vi "系统设置.vi"() -> ()   [LabVIEW 2016]
uses:
  <vilib>/Utility/miscctls.llb/LVPointTypeDef.ctl
  <userlib>/_SmartBalloon/Balloon Generic/Aesthetics.ctl
  <userlib>/_SmartBalloon/Balloon/Text Balloon.lvclass
  C:/Program Files (x86)/National Instruments/LabVIEW 2016/user.lib/_SmartBalloon/Balloon Generic/Balloon.lvclass
  <userlib>/_SmartBalloon/Balloon/Init Balloon.vi
  <vilib>/ptbypt/NI_PtbyPt.lvlib
  <vilib>/Utility/config.llb/NI_LVConfig.lvlib
  PLC/PLC.lvlib
  API/WxMessage/wxpusher.lvlib
  <userlib>/_SmartBalloon/API/SmartBalloon Library.lvclass
  <userlib>/_SmartBalloon/Balloon Generic/Balloon.lvclass
panel:
  in  "微信关注设置":bool
  in  "更新":bool
  in  "updateconfiguration":T1={"主机"="27.154.58.30", "用户"="update", "密码"="std23506", "远程路径"="数据传输系统\\平台数据传输系统.exe", "下载文件名"="平台数据传输系统.exe", "软件版本"=""}
  in  "自动运行启动参数":T2
  out "一级权限":bool
  in  "定时重启配置":bool
  in  "模块启用配置":bool
  in  "短信报警设置":bool
  in  "首页显示设置":bool
  in  "跨度核查":bool
  in  "空白核查":bool
  out "选项卡控件":enum32{"自由设定", "国标协议", "流量设定"}(tab)
  in  "24H周期设置":bool[](xcontrol)
  in  "运行间隔":i16=4 min=1 max=24
  in  "流量阈值":dbl=4.0 min=1.0 max=24.0
  in  "时间阈值":u16=4 min=1 max=24
  in  "周期设置":enum16{"自由设定", "国标协议", "流量设定"}(ring)
  out "二级权限":bool
  in  "质控启动日期":string(combo)="关闭"
  in  "跨度核查时间":u16(ring)=6 items=["00H", "01H", "02H", "03H", "04H", "05H", "06H", "07H", "08H", "09H", "10H", "11H", "12H", "13H", "14H", "15H", "16H", "17H", "18H", "19H", "20H", "21H", "22H", "23H", "关闭"]
  in  "空白核查时间":u16(ring)=2 items=["00H", "01H", "02H", "03H", "04H", "05H", "06H", "07H", "08H", "09H", "10H", "11H", "12H", "13H", "14H", "15H", "16H", "17H", "18H", "19H", "20H", "21H", "22H", "23H", "关闭"]
  in  "输入密码":u32
  out "布尔":bool
  in  "副屏显示设置":bool
  in  "开机启动":bool caption="氨氮禁用"
  in  "运行模式":enum16{"维护模式", "常规模式", "应急模式", "质控模式"}(ring)
  # "注：周期设置分为自由设定和国标协议两种。\n1：选择自由设定情况下：运行间隔将不可选用并变灰色，周期设置可自由手动勾选\n2：选择国标协议情况下：周期时间将由运行间隔选择的时间决定，下方周期设置被禁用并无法手动勾选。\n3：选择流量设定情况下：瞬时流量连续超过流量阈值到达时间阈值设定值，仪器将自动开启测量。"
  # "质控频次："
  # "零点核查时间："
  # "跨度核查时间："
  # "启动周期设置"
  # "m3/S"
  # "秒"
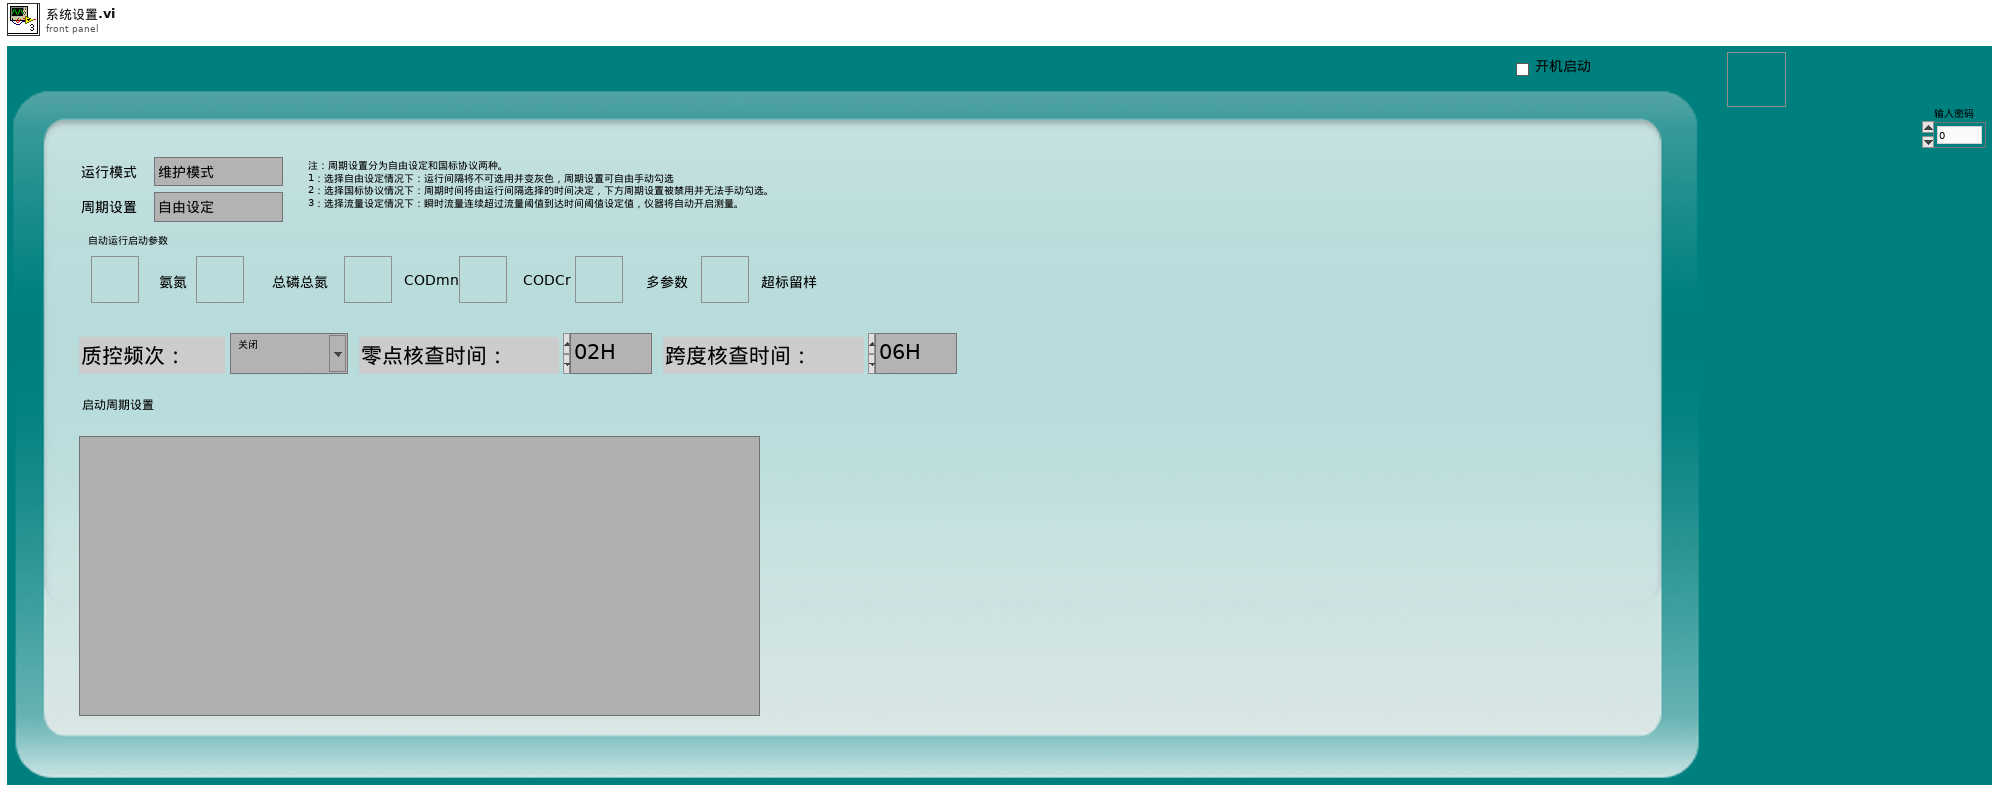
[diagram p1: front panel]
types:
  T1 = cluster{"主机":string, "用户":string, "密码":string, "远程路径":string, "下载文件名":string, "软件版本":string}
  T2 = cluster{"氨氮":bool, "总磷总氮":bool, "CODmn":bool, "CODCr":bool, "多参数":bool, "超标留样启用":bool}
  T3 = typedef "LVPointTypeDef.ctl" = cluster{"Horizontal":i16, "Vertical":i16}
  T4 = cluster{"频次":enum16{"关闭", "每天", "星期一", "星期二", "星期三", "星期四", "星期五", "星期六", "星期日"}, "时":u16, "分":u16}
  T5 = typedef "LVDateTimeRec.ctl" = cluster{"秒数的小数部分":dbl, "秒":i32, "分":i32, "时":i32, "日":i32, "月":i32, "年":i32, "天数（周）":i32, "天数（年）":i32, "DST":i32}
  T6 = enum16{"关闭", "每天", "星期一", "星期二", "星期三", "星期四", "星期五", "星期六", "星期日"}
  T7 = enum32{"Bad", "Idle", "Run top level", "Running"}
  T8 = typedef "NI_LVConfig.lvlib/Config Data RefNum.ctl" = refnum<k1>
  T9 = cluster{"运行模式":enum16{"维护模式", "常规模式", "应急模式", "质控模式"}}
  T10 = cluster{"测量模式":enum16{"水样测量", "标样核查", "零点核查", "跨度核查", "空白测试", "加标回收", "平行样", "校零", "校标"}}
  T11 = enum16{"启动测量", "标样核查", "零点核查", "跨度核查", "空白测试", "平行样测试", "加标回收", "空白校准", "标样校准", "初始化（清洗）", "停止测试", "仪器重启", "校时", "模式设置", "测量间隔设置"}
  T12 = cluster{"测试模式":enum16{"正常测试", "集成干预"}, "参数启用":cluster{"氨氮":bool, "总磷总氮":bool, "CODMn":bool, "CODcr":bool, "多参数":bool, "超标留样":bool}}
  T13 = cluster{"运行模式":enum16{"维护模式", "常规模式", "应急模式", "质控模式"}, "质控频次":enum16{"关闭", "每天", "星期一", "星期二", "星期三", "星期四", "星期五", "星期六", "星期日"}, "空白核查时间":u16, "跨度核查时间":u16, "24H周期设置":bool[]}
  T14 = enum32{"Invalid", "Standard", "Closed", "Hidden", "Minimized", "Maximized"}
  T15 = cluster{"氨氮":bool, "总磷总氮":bool, "CODmn":bool, "CODCr":bool, "多参数":bool, "超标留样":bool}
  T16 = typedef "Balloon Engine.lvlib/Balloon.lvclass/Aesthetics.ctl" = cluster{"Colors":cluster{"Font Color":u32, "Panel Color":u32}, "Display Time (ms)":i32}
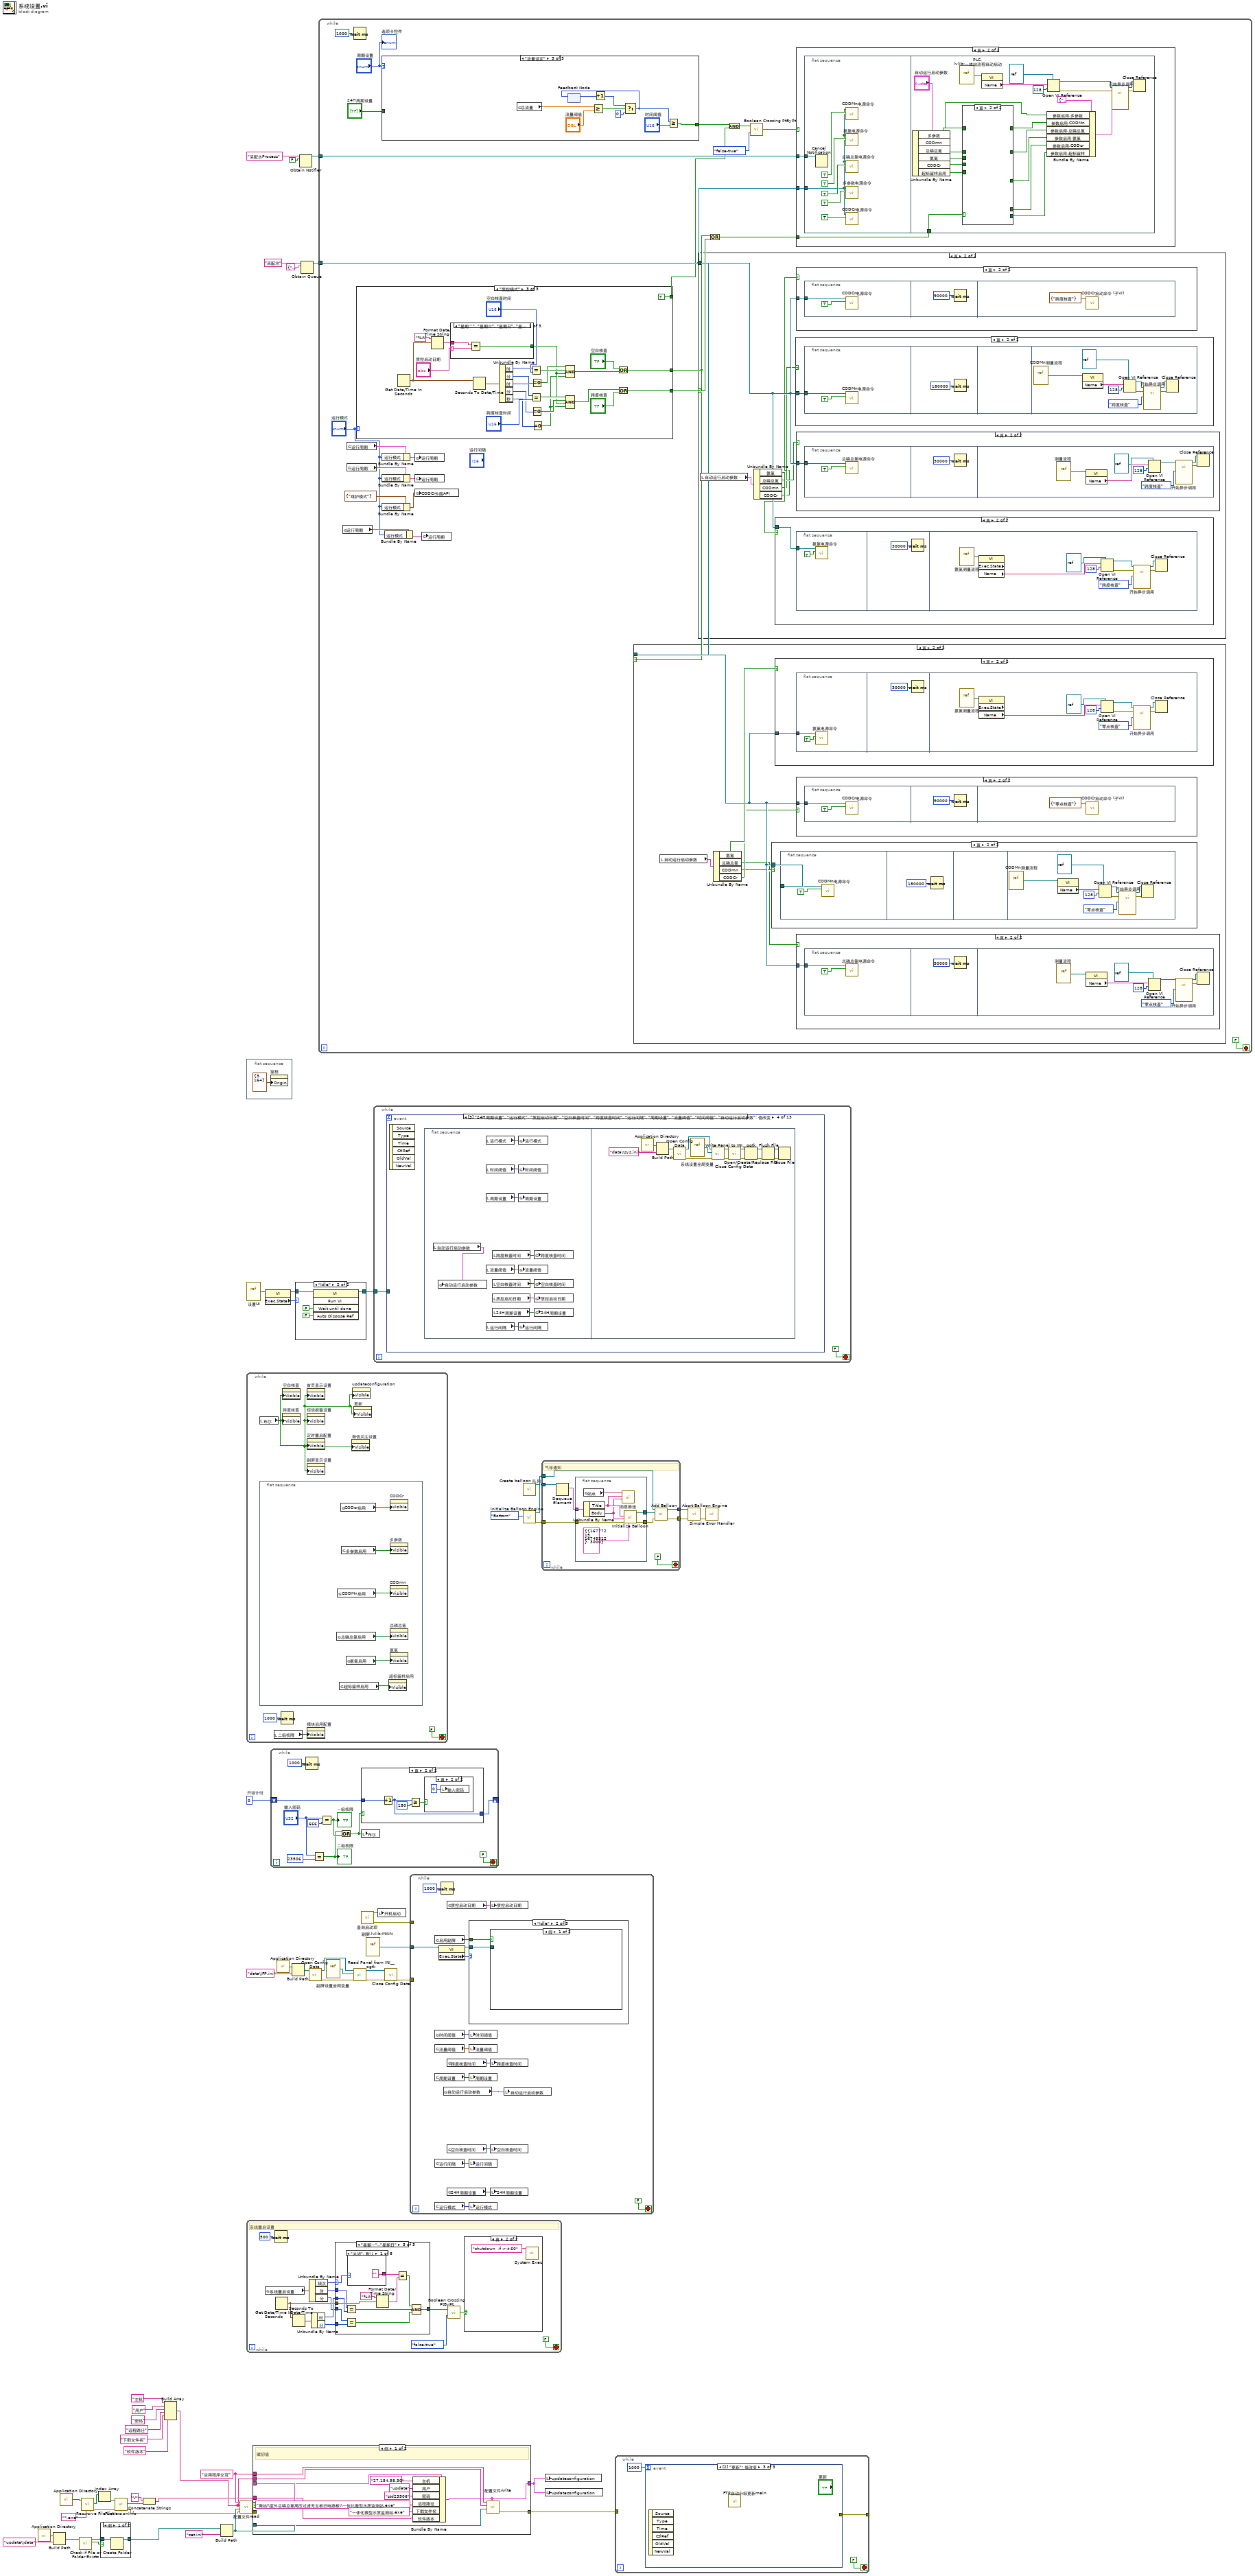
[diagram p0: block diagram]
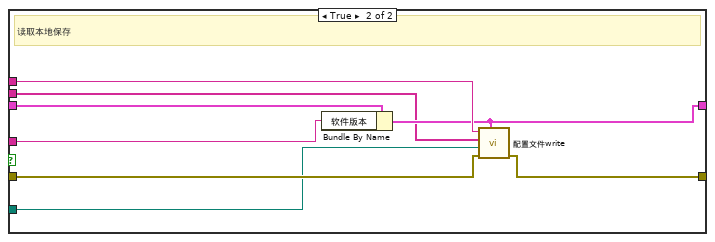
[diagram p3: hidden frame]
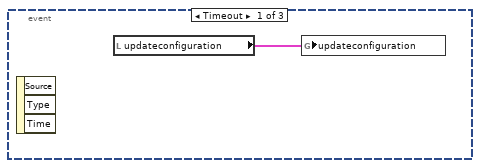
[diagram p4: hidden frame]
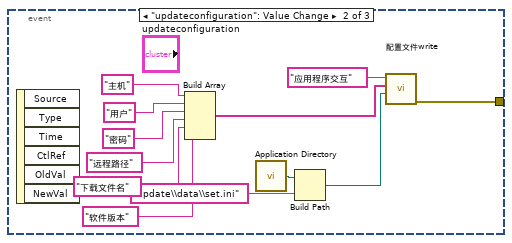
[diagram p5: hidden frame]
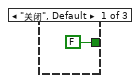
[diagram p7: hidden frame]
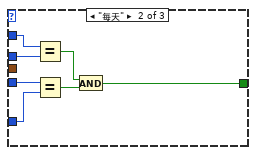
[diagram p8: hidden frame]
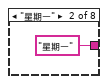
[diagram p9: hidden frame]
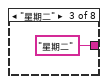
[diagram p10: hidden frame]
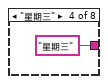
[diagram p11: hidden frame]
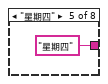
[diagram p12: hidden frame]
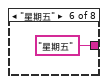
[diagram p13: hidden frame]
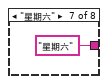
[diagram p14: hidden frame]
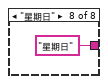
[diagram p15: hidden frame]
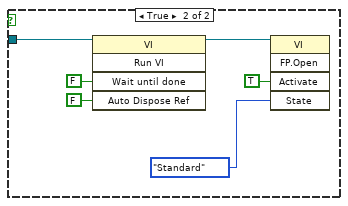
[diagram p20: hidden frame]
diagram:
  w35 = "应用程序交互" ("section")
  w56 = u32 0  # 开锁计时
  n1 = call <vilib>:"Application Directory.vi"() -> ("Application Directory"=w12:path)
  n2 = Build Path(base path=w12, name or relative path="update\\data" ("名称或相对路径")) -> (appended path=w13:path)
  n3 = call <vilib>:"Application Directory.vi"() -> ("Application Directory"=w30:path)
  n4 = call <vilib>:"Check if File or Folder Exists.vi"("path"=w13) -> ("file or folder exists?"=w14:bool, "dup path"=w15:path)  [unwired: 8 in, 1 out]
  n5 = call <vilib>:"Recursive File List.vi"("pattern"="*.exe", "Folder Path"=w30) -> ("error out"=w27:errorcluster, "All Files in Dir"=w29:path[])  [unwired: 5 in, 3 out]
  n6 = Index Array(array=w29) -> (element=w31:path)  [unwired: 1 in]
  n7 = case shown="假" w14 {
    tunnel: w15 -> [w62 w63]
    tunnel: [w61 w63] -> w10
    frame False {
      n8 = Create Folder(path (use dialog)=w62) -> (created path=w61:path)  [unwired: 2 in, 2 out]
    }
    frame True {
    }
  }
  n9 = call <vilib>:"FileVersionInfo.vi"("error in (no error)"=w27, "Application Path in"=w31) -> ("error out"=w24:errorcluster, "File Version Info"=w25:string)  [unwired: 6 in, 2 out]
  n10 = Concatenate Strings("V" ("字符串"), w25) -> (w23:string)
  n11 = Build Array("主机" ("section"), "用户" ("section"), "密码" ("key"), "远程路径" ("key"), "下载文件名" ("key"), "软件版本" ("key")) -> (w9:string[])
  n12 = Build Path(base path=w10, name or relative path="set.ini" ("名称或相对路径")) -> (appended path=w34:path)
  n13 = call "配置文件read.vi"("error in (no error)"=w24, "configuration file path"=w34, "键数组"=w9, "段"=w35) -> ("error out"=w33:errorcluster, "section exists?"=w36:bool, "updateconfiguration"=w32:T1)  [unwired: 5 in]
  n14 = flat-sequence {
    frame #0 {
      n15 = property on="窗格" class="Pane"("Origin"=T3 {"Horizontal"=3, "Vertical"=164} ("原点")) -> ()  [unwired: 2 in, 2 out]
    }
  }
  n16 = vi-ref "设置UI.vi"() -> (w51:refnum<vi>)
  n17 = while {
    stop <- FALSE stop-if-true
    n18 = local read "布尔"() -> (w65:bool)
    n19 = flat-sequence {
      frame #0 {
        n20 = global read "系统设置全局变量.vi" "总磷总氮启用"() -> (w70:bool)
        n21 = global read "系统设置全局变量.vi" "CODMn启用"() -> (w73:bool)
        n22 = global read "系统设置全局变量.vi" "超标留样启用"() -> (w69:bool)
        n23 = global read "系统设置全局变量.vi" "CODcr启用"() -> (w74:bool)
        n24 = global read "系统设置全局变量.vi" "多参数启用"() -> (w71:bool)
        n25 = global read "系统设置全局变量.vi" "氨氮启用"() -> (w72:bool)
        n26 = property on="超标留样启用" class="Bool (严格)"("Visible"=w69) -> ()  [unwired: 2 in, 2 out]
        n27 = property on="CODCr" class="Bool (严格)"("Visible"=w74) -> ()  [unwired: 2 in, 2 out]
        n28 = property on="多参数" class="Bool (严格)"("Visible"=w71) -> ()  [unwired: 2 in, 2 out]
        n29 = property on="CODmn" class="Bool (严格)"("Visible"=w73) -> ()  [unwired: 2 in, 2 out]
        n30 = property on="总磷总氮" class="Bool (严格)"("Visible"=w70) -> ()  [unwired: 2 in, 2 out]
        n31 = property on="氨氮" class="Bool (严格)"("Visible"=w72) -> ()  [unwired: 2 in, 2 out]
      }
    }
    n32 = local read "二级权限"() -> (w66:bool)
    n33 = Wait (ms)(milliseconds to wait=u32 1000 ("等待时间（毫秒）")) -> ()  [unwired: 1 out]
    n34 = property on="空白核查" class="Bool"("Visible"=w65) -> ()  [unwired: 2 in, 2 out]
    n35 = property on="跨度核查" class="Bool"("Visible"=w65) -> ()  [unwired: 2 in, 2 out]
    n36 = property on="首页显示设置" class="Bool"("Visible"=w65) -> ()  [unwired: 2 in, 2 out]
    n37 = property on="短信报警设置" class="Bool"("Visible"=w65) -> ()  [unwired: 2 in, 2 out]
    n38 = property on="定时重启配置" class="Bool"("Visible"=w65) -> ()  [unwired: 2 in, 2 out]
    n39 = property on="副屏显示设置" class="Bool"("Visible"=w65) -> ()  [unwired: 2 in, 2 out]
    n40 = property on="模块启用配置" class="Bool"("Visible"=w66) -> ()  [unwired: 2 in, 2 out]
    n41 = property on="微信关注设置" class="Bool"("Visible"=w65) -> ()  [unwired: 2 in, 2 out]
    n42 = property on="updateconfiguration" class="Clust (严格)"("Visible"=w65) -> ()  [unwired: 2 in, 2 out]
    n43 = property on="更新" class="Bool"("Visible"=w65) -> ()  [unwired: 2 in, 2 out]
  }
  n44 = while {
    stop <- FALSE stop-if-true
    # "系统重启设置"
    n45 = global read "系统设置全局变量.vi" "系统重启设置"() -> (w87:T4)
    n46 = Wait (ms)(milliseconds to wait=u32 500 ("等待时间（毫秒）")) -> ()  [unwired: 1 out]
    n47 = Get Date/Time In Seconds() -> (seconds since 1Jan1904=w78:timestamp)
    n48 = Seconds To Date/Time(time stamp (now)=w78) -> (date time rec=w85:T5)  [unwired: 1 in]
    n49 = Unbundle By Name(w87) -> ("频次"=w86:T6, "时"=w82:u16, "分"=w81:u16)
    n50 = Unbundle By Name(w85) -> ("时"=w84:i32, "分"=w83:i32)
    n51 = case shown="\"星期一\"..\"星期日\"" w86 {
      selector: w86 -> [_ _ w107]
      tunnel: [FALSE w90 w97] -> w77
      tunnel: w84 -> [_ w96 w101]
      tunnel: w83 -> [_ w93 w99]
      tunnel: w82 -> [_ w95 w102]
      tunnel: w81 -> [_ w94 w100]
      tunnel: w78 -> [_ _ w108]
      frame "关闭", Default {
      }
      frame "每天" {
        n52 = Equal?(x=w95, y=w96) -> (x = y?=w91:bool)
        n53 = Equal?(x=w94, y=w93) -> (x = y?=w92:bool)
        n54 = And(x=w91, y=w92) -> (x .and. y?=w90:bool)
      }
      frame "星期一".."星期日" {
        n55 = Equal?(x=w102, y=w101) -> (x = y?=w103:bool)
        n56 = Equal?(x=w100, y=w99) -> (x = y?=w104:bool)
        n57 = case shown="\"关闭\", 默认" w107 {
          tunnel: ["" ("时间格式字符串(%c)") "星期一" ("时间格式字符串(%c)") "星期二" ("时间格式字符串(%c)") "星期三" ("时间格式字符串(%c)") "星期四" ("时间格式字符串(%c)") "星期五" ("时间格式字符串(%c)") "星期六" ("时间格式字符串(%c)") "星期日" ("时间格式字符串(%c)")] -> w105
          frame "关闭", Default {
          }
          frame "星期一" {
          }
          frame "星期二" {
          }
          frame "星期三" {
          }
          frame "星期四" {
          }
          frame "星期五" {
          }
          frame "星期六" {
          }
          frame "星期日" {
          }
        }
        n58 = Format Date/Time String(time format string (%c)="%A" ("时间格式字符串(%c)"), seconds (now)=w108) -> (date/time string=w106:string)  [unwired: 1 in]
        n59 = Equal?(x=w105, y=w106) -> (x = y?=w98:bool)
        n60 = Compound Arithmetic op=AND ("复合运算")(w98, w103, w104) -> (w97:bool)
      }
    }
    n61 = call <vilib>:"Boolean Crossing PtByPt.vi"("direction"=enum16{"either", "false-true", "true-false"}."false-true", "input"=w77) -> ("crossing"=w75:bool)  [unwired: 1 in]
    n62 = case shown="真" w75 {
      frame False {
      }
      frame True {
        n63 = call <vilib>:"System Exec.vi"("command line"="shutdown  -f -r -t 60") -> ()  [unwired: 7 in, 4 out]
      }
    }
  }
  n64 = case shown="假" w36 {
    tunnel: w9 -> [w129 w133]
    tunnel: w35 -> [w128 w137]
    tunnel: w34 -> [w127 w131]
    tunnel: w33 -> [_ w132]
    tunnel: [w126 w130] -> w22
    tunnel: w32 -> [w120 w136]
    tunnel: [w118 w134] -> w8
    tunnel: w23 -> [w119 w135]
    frame False {
      # "赋初值"
      n65 = Bundle By Name(cluster=w120, "主机"="27.154.58.30" ("key"), "用户"="update", "密码"="std23506", "远程路径"="微站\\室外总磷总氮高压过滤无主板旧电路板\\一体化微型水质监测站.exe", "下载文件名"="一体化微型水质监测站.exe", "软件版本"=w119) -> (w118:T1)
      n66 = call "配置文件write.vi"("updateconfiguration"=w118, "configuration file path"=w127, "键数组"=w129, "段"=w128) -> ("error out"=w126:errorcluster)  [unwired: 7 in]
    }
    frame True {
      # "读取本地保存"
      n67 = Bundle By Name(cluster=w136, "软件版本"=w135) -> (w134:T1)
      n68 = call "配置文件write.vi"("updateconfiguration"=w134, "error in (no error)"=w132, "configuration file path"=w131, "键数组"=w133, "段"=w137) -> ("error out"=w130:errorcluster)  [unwired: 6 in]
    }
  }
  n69 = property class="VI"(reference=w51) -> (reference out=w49:refnum<vi>, "Exec.State"=w50:T7)  [unwired: 1 in, 1 out]
  n70 = while {
    shift-right: [w143] -> _
    shift-left: w56 -> [w144]
    stop <- FALSE stop-if-true
    n71 = Wait (ms)(milliseconds to wait=u32 1000 ("等待时间（毫秒）")) -> ()  [unwired: 1 out]
    n72 = Equal?(x="输入密码", y=u32 23506) -> (x = y?=w139:bool)
    "二级权限" <- w139
    n73 = Equal?(x="输入密码", y=u32 666) -> (x = y?=w140:bool)
    "一级权限" <- w140
    n74 = Or(x=w139, y=w140) -> (x .or. y?=w138:bool)
    n75 = case shown="真" w138 {
      tunnel: w144 -> [_ w151]
      tunnel: [_ w150] -> w143
      frame False {
      }
      frame True {
        n76 = Increment(x=w151) -> (x+1=w150:u32)
        n77 = Greater Or Equal?(x=w150, y=u32 180) -> (x >= y?=w148:bool)
        n78 = case shown="真" w148 {
          frame False {
          }
          frame True {
            n79 = local write "输入密码"(u32 0 ("输入密码")) -> ()
          }
        }
      }
    }
    n80 = local write "布尔"(w138) -> ()
  }
  n81 = call <vilib>:"Application Directory.vi"() -> ("Application Directory"=w38:path)
  n82 = Build Path(base path=w38, name or relative path="data\\FP.ini" ("名称或相对路径")) -> (appended path=w45:path)
  n83 = case shown="\"Idle\"" w50 {
    tunnel: w49 -> [w153 w157]
    tunnel: [w153 w156] -> w48
    frame "Bad", Default {
    }
    frame "Idle" {
      n84 = invoke class="VI" method="Run VI"(reference=w157, "Wait until done"=FALSE ("结束前等待"), "Auto Dispose Ref"=FALSE ("自动销毁引用")) -> (reference out=w156:refnum<vi>)  [unwired: 2 in, 4 out]
    }
  }
  n85 = Obtain Notifier(name (unnamed)="采配水Process" ("名称（未命名）"), notification data type=FALSE) -> (notifier out=w58:refnum<notifier>)  [unwired: 2 in, 2 out]
  n86 = Obtain Queue(name (unnamed)="采配水" ("名称（未命名）"), element data type=cluster{"命令":string, "数据":variant} {"命令"="", "数据"=variant}) -> (queue out=w53:refnum<queue>)  [unwired: 3 in, 2 out]
  n87 = call <vilib>:"Open Config Data.vi"("configuration file path"=w45) -> ("error out"=w44:errorcluster, "refnum"=w41:T8)  [unwired: 8 in, 1 out]
  n88 = while {
    tunnel: w58 -> [w178]
    tunnel: w53 -> [w174]
    stop <- FALSE stop-if-true
    n89 = global read "CODMn断电保存全局变量.vi" "运行周期"() -> (w160:T13)
    n90 = global read "氨氮断电保存全局变量.vi" "运行周期"() -> (w164:T13)
    n91 = global read "总磷总氮断电保存全局变量.vi" "运行周期"() -> (w162:T13)
    n92 = Wait (ms)(milliseconds to wait=u32 1000 ("等待时间（毫秒）")) -> ()  [unwired: 1 out]
    n93 = case shown="\"质控模式\"" "运行模式" {
      tunnel: [_ _ w351] -> w167
      tunnel: [_ _ w355] -> w166
      tunnel: [_ TRUE TRUE] -> w171
      frame "维护模式", Default {
      }
      frame "常规模式" {
      }
      frame "质控模式" {
        n94 = Get Date/Time In Seconds() -> (seconds since 1Jan1904=w362:timestamp)
        n95 = Format Date/Time String(time format string (%c)="%A" ("时间格式字符串(%c)"), seconds (now)=w362) -> (date/time string=w360:string)  [unwired: 1 in]
        n96 = case shown="\"星期二\", \"星期六\", \"星期日\", \"星期三\", \"星期四\", \"星期五\", \"星期一\"" "质控启动日期" {
          selector: "质控启动日期" -> [w378 _ _]
          tunnel: [w377 TRUE FALSE] -> w363
          tunnel: w360 -> [w376 _ _]
          frame "星期二", "星期六", "星期日", "星期三", "星期四", "星期五", "星期一" {
            n97 = Equal?(x=w376, y=w378) -> (x = y?=w377:bool)
          }
          frame "每天" {
          }
          frame "关闭", Default {
          }
        }
        n98 = Seconds To Date/Time(time stamp (now)=w362) -> (date time rec=w375:T5)  [unwired: 1 in]
        n99 = Unbundle By Name(w375) -> ("时"=w374:i32, "分"=w372:i32, "时"=w368:i32, "分"=w367:i32, "秒"=w359:i32)
        n100 = Equal?(x=w374, y="空白核查时间") -> (x = y?=w371:bool)
        n101 = Equal?(x=w368, y="跨度核查时间") -> (x = y?=w366:bool)
        n102 = Equal To 0?(x=w372) -> (x = 0?=w370:bool)
        n103 = Equal To 0?(x=w367) -> (x = 0?=w365:bool)
        n104 = Equal To 0?(x=w359) -> (x = 0?=w358:bool)
        n105 = Compound Arithmetic op=AND ("复合运算")(w370, w371, w363, w358) -> (w356:bool)
        n106 = Compound Arithmetic op=AND ("复合运算")(w366, w365, w363, w358) -> (w353:bool)
        n107 = Or(x="空白核查", y=w356) -> (x .or. y?=w355:bool)
        n108 = Or(x=w353, y="跨度核查") -> (x .or. y?=w351:bool)
      }
    }
    n109 = case shown="\"流量设定\"" "周期设置" {
      tunnel: [w182 w189 w205] -> w170
      tunnel: "24H周期设置" -> [w181 w190 _]
      frame "自由设定", Default {
        n110 = Get Date/Time In Seconds() -> (seconds since 1Jan1904=w183:timestamp)
        n111 = Seconds To Date/Time(time stamp (now)=w183) -> (date time rec=w184:T5)  [unwired: 1 in]
        n112 = Unbundle By Name(w184) -> ("时"=w187:i32, "分"=w185:i32)
        n113 = Index Array(array=w181, index=w187) -> (element=w188:bool)
        n114 = Equal To 0?(x=w185) -> (x = 0?=w186:bool)
        n115 = And(x=w188, y=w186) -> (x .and. y?=w182:bool)
      }
      frame "国标协议" {
        n116 = Get Date/Time In Seconds() -> (seconds since 1Jan1904=w191:timestamp)
        n117 = local read "运行间隔"() -> (w200:i16)
        n118 = Seconds To Date/Time(time stamp (now)=w191) -> (date time rec=w192:T5)  [unwired: 1 in]
        n119 = call "运行间隔计算.vi"("运行周期"=w200) -> ("数组"=w199:i32[])  [unwired: 10 in]
        n120 = Unbundle By Name(w192) -> ("时"=w195:i32, "分"=w193:i32)
        n121 = Index Array(array=w190, index=w195) -> (element=w196:bool)
        n122 = Equal To 0?(x=w193) -> (x = 0?=w194:bool)
        n123 = And(x=w196, y=w194) -> (x .and. y?=w189:bool)
        n124 = for {
          tunnel: w199 -> [w203] mode=indexing
          shift-right: [w201] -> w197
          shift-left: bool[] [FALSE, FALSE, FALSE, FALSE, FALSE, FALSE, FALSE, FALSE, FALSE, FALSE, FALSE, FALSE, FALSE, FALSE, FALSE, FALSE, FALSE, FALSE, FALSE, FALSE, FALSE, FALSE, FALSE, FALSE] ("24H周期设置") -> [w204]
          n125 = Replace Array Subset(array=w204, new element=TRUE ("新元素/子数组"), index=w203) -> (w201:bool[])
        }
        n126 = local write "24H周期设置"(w197) -> ()
        n127 = global write "系统设置全局变量.vi" "24H周期设置"(w197) -> ()
      }
      frame "流量设定" {
        n128 = global read "流量计全局变量.vi" "总流量"() -> (w213:dbl)
        n129 = feedback #1() -> (w210:i16)  [unwired: 1 in]
        n130 = Greater Or Equal?(x=w213, y="流量阈值") -> (x >= y?=w208:bool)
        n131 = Increment(x=w210) -> (x+1=w209:i16)
        n132 = Select(t=w209, s=w208, f=i16 0) -> (s? t:f=w207:i16)
        n133 = feedback-in #1(w207) -> ()
        n134 = Greater Or Equal?(x=w207, y="时间阈值") -> (x >= y?=w205:bool)
      }
    }
    n135 = Bundle By Name(cluster=w164, "运行模式"="运行模式") -> (w163:T13)
    n136 = Bundle By Name(cluster=w162, "运行模式"="运行模式") -> (w161:T13)
    n137 = Bundle By Name(cluster=T9 {"运行模式"=enum."维护模式"} ("外围API"), "运行模式"="运行模式") -> (w168:T9)
    n138 = Bundle By Name(cluster=w160, "运行模式"="运行模式") -> (w158:T13)
    n139 = global write "氨氮断电保存全局变量.vi" "运行周期"(w163) -> ()
    n140 = global write "总磷总氮断电保存全局变量.vi" "运行周期"(w161) -> ()
    n141 = global write "CODCr外部API.vi" "CODCr外围API"(w168) -> ()
    n142 = global write "CODMn断电保存全局变量.vi" "运行周期"(w158) -> ()
    n143 = case shown="真" w166 {
      tunnel: w174 -> [_ w268]
      frame False {
      }
      frame True {
        n144 = local read "自动运行启动参数"() -> (w267:T2)
        n145 = Unbundle By Name(w267) -> ("氨氮"=w266:bool, "总磷总氮"=w263:bool, "CODmn"=w264:bool, "CODCr"=w265:bool)
        n146 = case shown="真" w264 {
          tunnel: w268 -> [_ w274]
          frame False {
          }
          frame True {
            n147 = flat-sequence {
              tunnel: w274 -> [w275]
              frame #0 {
                n148 = call "CODMn电源命令.vi"("通电/断电"=TRUE, "队列"=w275) -> ()  [unwired: 9 in, 1 out]
              }
              frame #1 {
                n149 = Wait (ms)(milliseconds to wait=u32 180000 ("等待时间（毫秒）")) -> ()  [unwired: 1 out]
              }
              frame #2 {
              }
              frame #3 {
                n150 = vi-ref "CODMn测量流程.vi"() -> (w285:refnum<vi>)
                n151 = property class="VI"(reference=w285) -> ("Name"=w286:string)  [unwired: 1 in, 2 out]
                n152 = Open VI Reference(type specifier VI Refnum (for type only)=refnum<vi> refnum, vi path=w286, options=128 ("选项")) -> (vi reference=w280:refnum<vi>, error out=w282:errorcluster)  [unwired: 3 in]
                n153 = call-by-ref "开始异步调用"(reference=w280, error in=w282, "控制命令"=T11."零点核查") -> (reference out=w283:refnum<vi>, error out=w284:errorcluster)  [unwired: 11 in]
                n154 = Close Reference(reference=w283, error in (no error)=w284) -> ()  [unwired: 1 out]
              }
            }
          }
        }
        n155 = case shown="真" w266 {
          tunnel: w268 -> [_ w299]
          frame False {
          }
          frame True {
            n156 = flat-sequence {
              tunnel: w299 -> [w300]
              frame #0 {
                n157 = call "氨氮电源命令.vi"("通电/断电"=TRUE, "队列"=w300) -> ()  [unwired: 9 in, 1 out]
              }
              frame #1 {
                n158 = Wait (ms)(milliseconds to wait=u32 30000 ("等待时间（毫秒）")) -> ()  [unwired: 1 out]
              }
              frame #2 {
                n159 = vi-ref "氨氮测量流程.vi"() -> (w311:refnum<vi>)
                n160 = property class="VI" props=["Exec.State", "Name"](reference=w311) -> ("Name"=w310:string)  [unwired: 1 in, 3 out]
                n161 = Open VI Reference(type specifier VI Refnum (for type only)=refnum<vi> refnum, vi path=w310, options=128 ("选项")) -> (vi reference=w305:refnum<vi>, error out=w307:errorcluster)  [unwired: 3 in]
                n162 = call-by-ref "开始异步调用"(reference=w305, error in=w307, "控制命令"=T11."零点核查") -> (reference out=w308:refnum<vi>, error out=w309:errorcluster)  [unwired: 11 in]
                n163 = Close Reference(reference=w308, error in (no error)=w309) -> ()  [unwired: 1 out]
              }
            }
          }
        }
        n164 = case shown="真" w265 {
          tunnel: w268 -> [_ w269]
          frame False {
          }
          frame True {
            n165 = flat-sequence {
              tunnel: w269 -> [w270]
              frame #0 {
                n166 = call "CODCr电源命令.vi"("通电/断电"=TRUE, "队列"=w270) -> ()  [unwired: 9 in, 1 out]
              }
              frame #1 {
                n167 = Wait (ms)(milliseconds to wait=u32 90000 ("等待时间（毫秒）")) -> ()  [unwired: 1 out]
              }
              frame #2 {
                n168 = call "CODCr启动命令 (子VI).vi"("启动测量模式"=T10 {"测量模式"=enum."零点核查"}) -> ()  [unwired: 11 in]
              }
            }
          }
        }
        n169 = case shown="真" w263 {
          tunnel: w268 -> [_ w287]
          frame False {
          }
          frame True {
            n170 = flat-sequence {
              tunnel: w287 -> [w289]
              frame #0 {
                n171 = call "总磷总氮电源命令.vi"("通电/断电"=TRUE, "队列"=w289) -> ()  [unwired: 9 in, 1 out]
              }
              frame #1 {
                n172 = Wait (ms)(milliseconds to wait=u32 30000 ("等待时间（毫秒）")) -> ()  [unwired: 1 out]
              }
              frame #2 {
                n173 = vi-ref "测量流程.vi"() -> (w296:refnum<vi>)
                n174 = property class="VI"(reference=w296) -> ("Name"=w297:string)  [unwired: 1 in, 2 out]
                n175 = Open VI Reference(type specifier VI Refnum (for type only)=refnum<vi> refnum, vi path=w297, options=128 ("选项")) -> (vi reference=w295:refnum<vi>)  [unwired: 3 in, 1 out]
                n176 = call-by-ref "开始异步调用"(reference=w295, "控制命令"=T11."零点核查") -> (reference out=w294:refnum<vi>, error out=w293:errorcluster)  [unwired: 12 in]
                n177 = Close Reference(reference=w294, error in (no error)=w293) -> ()  [unwired: 1 out]
              }
            }
          }
        }
      }
    }
    n178 = case shown="真" w167 {
      tunnel: w174 -> [_ w219]
      frame False {
      }
      frame True {
        n179 = local read "自动运行启动参数"() -> (w218:T2)
        n180 = Unbundle By Name(w218) -> ("氨氮"=w217:bool, "总磷总氮"=w216:bool, "CODmn"=w215:bool, "CODCr"=w214:bool)
        n181 = case shown="真" w217 {
          tunnel: w219 -> [_ w250]
          frame False {
          }
          frame True {
            n182 = flat-sequence {
              tunnel: w250 -> [w251]
              frame #0 {
                n183 = call "氨氮电源命令.vi"("通电/断电"=TRUE, "队列"=w251) -> ()  [unwired: 9 in, 1 out]
              }
              frame #1 {
                n184 = Wait (ms)(milliseconds to wait=u32 30000 ("等待时间（毫秒）")) -> ()  [unwired: 1 out]
              }
              frame #2 {
                n185 = vi-ref "氨氮测量流程.vi"() -> (w262:refnum<vi>)
                n186 = property class="VI" props=["Exec.State", "Name"](reference=w262) -> ("Name"=w261:string)  [unwired: 1 in, 3 out]
                n187 = Open VI Reference(type specifier VI Refnum (for type only)=refnum<vi> refnum, vi path=w261, options=128 ("选项")) -> (vi reference=w256:refnum<vi>, error out=w258:errorcluster)  [unwired: 3 in]
                n188 = call-by-ref "开始异步调用"(reference=w256, error in=w258, "控制命令"=T11."跨度核查") -> (reference out=w259:refnum<vi>, error out=w260:errorcluster)  [unwired: 11 in]
                n189 = Close Reference(reference=w259, error in (no error)=w260) -> ()  [unwired: 1 out]
              }
            }
          }
        }
        n190 = case shown="真" w215 {
          tunnel: w219 -> [_ w225]
          frame False {
          }
          frame True {
            n191 = flat-sequence {
              tunnel: w225 -> [w226]
              frame #0 {
                n192 = call "CODMn电源命令.vi"("通电/断电"=TRUE, "队列"=w226) -> ()  [unwired: 9 in, 1 out]
              }
              frame #1 {
                n193 = Wait (ms)(milliseconds to wait=u32 180000 ("等待时间（毫秒）")) -> ()  [unwired: 1 out]
              }
              frame #2 {
              }
              frame #3 {
                n194 = vi-ref "CODMn测量流程.vi"() -> (w236:refnum<vi>)
                n195 = property class="VI"(reference=w236) -> ("Name"=w237:string)  [unwired: 1 in, 2 out]
                n196 = Open VI Reference(type specifier VI Refnum (for type only)=refnum<vi> refnum, vi path=w237, options=128 ("选项")) -> (vi reference=w231:refnum<vi>, error out=w233:errorcluster)  [unwired: 3 in]
                n197 = call-by-ref "开始异步调用"(reference=w231, error in=w233, "控制命令"=T11."跨度核查") -> (reference out=w234:refnum<vi>, error out=w235:errorcluster)  [unwired: 11 in]
                n198 = Close Reference(reference=w234, error in (no error)=w235) -> ()  [unwired: 1 out]
              }
            }
          }
        }
        n199 = case shown="真" w214 {
          tunnel: w219 -> [_ w220]
          frame False {
          }
          frame True {
            n200 = flat-sequence {
              tunnel: w220 -> [w221]
              frame #0 {
                n201 = call "CODCr电源命令.vi"("通电/断电"=TRUE, "队列"=w221) -> ()  [unwired: 9 in, 1 out]
              }
              frame #1 {
                n202 = Wait (ms)(milliseconds to wait=u32 90000 ("等待时间（毫秒）")) -> ()  [unwired: 1 out]
              }
              frame #2 {
                n203 = call "CODCr启动命令 (子VI).vi"("启动测量模式"=T10 {"测量模式"=enum."跨度核查"}) -> ()  [unwired: 11 in]
              }
            }
          }
        }
        n204 = case shown="真" w216 {
          tunnel: w219 -> [_ w238]
          frame False {
          }
          frame True {
            n205 = flat-sequence {
              tunnel: w238 -> [w240]
              frame #0 {
                n206 = call "总磷总氮电源命令.vi"("通电/断电"=TRUE, "队列"=w240) -> ()  [unwired: 9 in, 1 out]
              }
              frame #1 {
                n207 = Wait (ms)(milliseconds to wait=u32 30000 ("等待时间（毫秒）")) -> ()  [unwired: 1 out]
              }
              frame #2 {
                n208 = vi-ref "测量流程.vi"() -> (w247:refnum<vi>)
                n209 = property class="VI"(reference=w247) -> ("Name"=w248:string)  [unwired: 1 in, 2 out]
                n210 = Open VI Reference(type specifier VI Refnum (for type only)=refnum<vi> refnum, vi path=w248, options=128 ("选项")) -> (vi reference=w246:refnum<vi>)  [unwired: 3 in, 1 out]
                n211 = call-by-ref "开始异步调用"(reference=w246, "控制命令"=T11."跨度核查") -> (reference out=w245:refnum<vi>, error out=w244:errorcluster)  [unwired: 12 in]
                n212 = Close Reference(reference=w245, error in (no error)=w244) -> ()  [unwired: 1 out]
              }
            }
          }
        }
      }
    }
    n213 = Or(x=w166, y=w167) -> (x .or. y?=w165:bool)
    n214 = And(x=w170, y=w171) -> (x .and. y?=w169:bool)
    n215 = call <vilib>:"Boolean Crossing PtByPt.vi"("direction"=enum16{"either", "false-true", "true-false"}."false-true", "input"=w169) -> ("crossing"=w176:bool)  [unwired: 1 in]
    n216 = case shown="真" w176 {
      tunnel: w178 -> [_ w314]
      tunnel: w174 -> [_ w313]
      tunnel: w165 -> [_ w312]
      frame False {
      }
      frame True {
        n217 = flat-sequence {
          tunnel: w314 -> [w321]
          tunnel: w313 -> [w315]
          tunnel: w312 -> [w332]
          frame #0 {
            n218 = Cancel Notification(0:w321) -> ()  [unwired: 1 in, 3 out]
            n219 = call "CODMn电源命令.vi"("通电/断电"=TRUE, "队列"=w315) -> ()  [unwired: 9 in, 1 out]
            n220 = call "氨氮电源命令.vi"("通电/断电"=TRUE, "队列"=w315) -> ()  [unwired: 9 in, 1 out]
            n221 = call "总磷总氮电源命令.vi"("通电/断电"=TRUE, "队列"=w315) -> ()  [unwired: 9 in, 1 out]
            n222 = call "多参数电源命令.vi"("通电/断电"=TRUE, "队列"=w315) -> ()  [unwired: 9 in, 1 out]
            n223 = call "CODCr电源命令.vi"("通电/断电"=TRUE, "队列"=w315) -> ()  [unwired: 9 in, 1 out]
          }
          frame #1 {
            n224 = Unbundle By Name("自动运行启动参数") -> ("多参数"=w326:bool, "CODmn"=w327:bool, "总磷总氮"=w328:bool, "氨氮"=w329:bool, "CODCr"=w330:bool, "超标留样启用"=w322:bool)
            n225 = vi-ref "PLC.lvlib:一体站流程自动启动.vi"() -> (w338:refnum<vi>)
            n226 = case shown="真" w332 {
              tunnel: [w346 _] -> w344
              tunnel: [w347 _] -> w343
              tunnel: [w349 _] -> w342
              tunnel: [w348 _] -> w341
              tunnel: w330 -> [w349 _]
              tunnel: w329 -> [w348 _]
              tunnel: w328 -> [w347 _]
              tunnel: w327 -> [w346 _]
              tunnel: [w345 _] -> w323
              tunnel: w322 -> [w345 _]
              frame False {
              }
              frame True {
              }
            }
            n227 = property class="VI"(reference=w338) -> ("Name"=w339:string)  [unwired: 1 in, 2 out]
            n228 = Bundle By Name(cluster=T12 {"测试模式"=enum."正常测试", "参数启用"={"氨氮"=FALSE, "总磷总氮"=FALSE, "CODMn"=FALSE, "CODcr"=FALSE, "多参数"=FALSE, "超标留样"=FALSE}} ("参数"), "参数启用.多参数"=w326, "参数启用.CODMn"=w344, "参数启用.总磷总氮"=w343, "参数启用.氨氮"=w341, "参数启用.CODcr"=w342, "参数启用.超标留样"=w323) -> (w324:T12)
            n229 = Open VI Reference(type specifier VI Refnum (for type only)=refnum<vi> refnum, vi path=w339, options=128 ("选项")) -> (vi reference=w337:refnum<vi>, error out=w336:errorcluster)  [unwired: 3 in]
            n230 = call-by-ref "开始异步调用"(reference=w337, error in=w336, "参数"=w324) -> (reference out=w335:refnum<vi>, error out=w334:errorcluster)  [unwired: 11 in]
            n231 = Close Reference(reference=w335, error in (no error)=w334) -> ()  [unwired: 1 out]
          }
        }
      }
    }
    "选项卡控件" <- "周期设置"
  }
  n232 = vi-ref "副屏设置全局变量.vi"() -> (w42:refnum<vi>)
  n233 = call <userlib>:"Read Panel from INI__ogtk.vi"("error in (no error)"=w44, "VI ref"=w42, "refnum"=w41) -> ("error out"=w43:errorcluster, "refnum out"=w40:T8)  [unwired: 7 in]
  n234 = call "查询启动项.vi"() -> ("error out"=w47:errorcluster, "包含启动项"=w57:bool)  [unwired: 10 in]
  n235 = vi-ref "副屏.lvlib:MAIN.vi"() -> (w52:refnum<vi>)
  n236 = while {
    tunnel: w48 -> [w381]
    stop <- FALSE stop-if-true
    n237 = event shown="[3] \"24H周期设置\", \"运行模式\", \"质控启动日期\", \"空白核查时间\", \"跨度核查时间\", \"运行间隔\", \"周期设置\", \"流量阈值\", \"时间阈值\", \"自动运行启动参数\": 值改变" {
      selector: _ -> [_ _ _ _ _ _ _ _ _ _ _ _ _]
      dyn-events: _ -> [_ _ _ _ _ _ _ _ _ _ _ _ _]
      timeout: _ -> [_ _ _ _ _ _ _ _ _ _ _ _ _]
      tunnel: w381 -> [_ _ _ _ _ _ _ _ _ _ w428 _ _]
      event Timeout {
        n238 = event-data() -> ()  [unwired: 1 in, 3 out]
      }
      event "定时重启配置": Value Change {
        n239 = event-data() -> ()  [unwired: 1 in, 6 out]
        n240 = call "重启设置.vi"() -> ()  [unwired: 12 in]
      }
      event "模块启用配置": Value Change {
        n241 = event-data() -> ()  [unwired: 1 in, 6 out]
        n242 = call "模块启用配置框.vi"() -> ()  [unwired: 12 in]
      }
      event "24H周期设置", "运行模式", "质控启动日期", "空白核查时间", "跨度核查时间", "运行间隔", "周期设置", "流量阈值", "时间阈值", "自动运行启动参数": Value Change {
        n243 = event-data() -> ()  [unwired: 1 in, 6 out]
        n244 = flat-sequence {
          frame #0 {
            n245 = local read "自动运行启动参数"() -> (w383:T2)
            n246 = global write "系统设置全局变量.vi" "自动运行启动参数"(w383) -> ()
            n247 = local read "运行模式"() -> (w392:enum16{"维护模式", "常规模式", "应急模式", "质控模式"})
            n248 = local read "时间阈值"() -> (w385:u16)
            n249 = local read "周期设置"() -> (w386:enum16{"自由设定", "国标协议", "流量设定"})
            n250 = local read "流量阈值"() -> (w384:dbl)
            n251 = local read "运行间隔"() -> (w387:i16)
            n252 = local read "跨度核查时间"() -> (w388:u16)
            n253 = local read "空白核查时间"() -> (w389:u16)
            n254 = local read "质控启动日期"() -> (w390:string)
            n255 = local read "24H周期设置"() -> (w391:bool[])
            n256 = global write "系统设置全局变量.vi" "运行模式"(w392) -> ()
            n257 = global write "系统设置全局变量.vi" "时间阈值"(w385) -> ()
            n258 = global write "系统设置全局变量.vi" "周期设置"(w386) -> ()
            n259 = global write "系统设置全局变量.vi" "流量阈值"(w384) -> ()
            n260 = global write "系统设置全局变量.vi" "运行间隔"(w387) -> ()
            n261 = global write "系统设置全局变量.vi" "跨度核查时间"(w388) -> ()
            n262 = global write "系统设置全局变量.vi" "空白核查时间"(w389) -> ()
            n263 = global write "系统设置全局变量.vi" "质控启动日期"(w390) -> ()
            n264 = global write "系统设置全局变量.vi" "24H周期设置"(w391) -> ()
          }
          frame #1 {
            n265 = call <vilib>:"Application Directory.vi"() -> ("Application Directory"=w406:path)
            n266 = Build Path(base path=w406, name or relative path="data\\sys.ini" ("名称或相对路径")) -> (appended path=w404:path)
            n267 = call <vilib>:"Open Config Data.vi"("configuration file path"=w404) -> ("error out"=w400:errorcluster, "refnum"=w403:T8)  [unwired: 8 in, 1 out]
            n268 = vi-ref "系统设置全局变量.vi"() -> (w402:refnum<vi>)
            n269 = call <userlib>:"Write Panel to INI__ogtk.vi"("error in (no error)"=w400, "VI ref"=w402, "refnum"=w403) -> ("error out"=w399:errorcluster, "refnum out"=w401:T8)  [unwired: 7 in]
            n270 = call <vilib>:"Close Config Data.vi"("error in (no error)"=w399, "refnum"=w401) -> ("error out"=w394:errorcluster, "file path"=w393:path)  [unwired: 8 in]
            n271 = Open/Create/Replace File(file path (use dialog)=w393, error in=w394) -> (refnum out=w397:refnum<file>, error out=w398:errorcluster)  [unwired: 4 in, 1 out]
            n272 = Flush File(refnum=w397, error in=w398) -> (refnum out=w396:refnum<file>, error out=w395:errorcluster)
            n273 = Close File(refnum=w396, error in=w395) -> ()  [unwired: 2 out]
          }
        }
      }
      event "运行间隔": Mouse Down {
        n274 = event-data() -> ("CtlRef"=w410:refnum<vi>)  [unwired: 1 in, 7 out]
        n275 = property class="DigNum (严格)"(reference=w410) -> (reference out=w409:refnum<vi>, "Value"=w408:i16)  [unwired: 1 in, 1 out]
        n276 = call "数字键盘.vi"("OldNumber"=w408) -> ("NewNumber"=w407:sgl)
        n277 = property class="DigNum (严格)"(reference=w409, "Val(Sgnl)"=w407) -> ()  [unwired: 1 in, 2 out]
      }
      event "流量阈值": Mouse Down {
        n278 = event-data() -> ("CtlRef"=w414:refnum<vi>)  [unwired: 1 in, 7 out]
        n279 = property class="DigNum (严格)"(reference=w414) -> (reference out=w413:refnum<vi>, "Value"=w412:dbl)  [unwired: 1 in, 1 out]
        n280 = call "数字键盘.vi"("OldNumber"=w412) -> ("NewNumber"=w411:sgl)
        n281 = property class="DigNum (严格)"(reference=w413, "Val(Sgnl)"=w411) -> ()  [unwired: 1 in, 2 out]
      }
      event "时间阈值": Mouse Down {
        n282 = event-data() -> ("CtlRef"=w418:refnum<vi>)  [unwired: 1 in, 7 out]
        n283 = property class="DigNum (严格)"(reference=w418) -> (reference out=w417:refnum<vi>, "Value"=w416:u16)  [unwired: 1 in, 1 out]
        n284 = call "数字键盘.vi"("OldNumber"=w416) -> ("NewNumber"=w415:sgl)
        n285 = property class="DigNum (严格)"(reference=w417, "Val(Sgnl)"=w415) -> ()  [unwired: 1 in, 2 out]
      }
      event "开机启动": Value Change {
        n286 = event-data() -> ("NewVal"=w419:bool)  [unwired: 1 in, 5 out]
        n287 = case shown="假" w419 {
          frame False {
            n288 = call "删除启动项.vi"() -> ("删除标记"=w420:bool)  [unwired: 10 in, 1 out]
            n289 = case shown="假" w420 {
              frame False {
                n290 = local write "开机启动"(TRUE ("开机启动")) -> ()
                n291 = One Button Dialog(message="启动项删除失败" ("消息")) -> ()  [unwired: 1 in, 1 out]
              }
              frame True {
              }
            }
          }
          frame True {
            n292 = call "添加启动项.vi"() -> ("添加成功标记"=w423:bool)  [unwired: 10 in, 1 out]
            n293 = case shown="假" w423 {
              frame False {
                n294 = local write "开机启动"(FALSE ("开机启动")) -> ()
                n295 = One Button Dialog(message="启动项添加失败" ("消息")) -> ()  [unwired: 1 in, 1 out]
              }
              frame True {
              }
            }
          }
        }
      }
      event "副屏显示设置": Value Change {
        n296 = event-data() -> ()  [unwired: 1 in, 6 out]
        n297 = call "副屏设置.vi"() -> ()  [unwired: 12 in]
      }
      event "首页显示设置": Value Change {
        n298 = event-data() -> ()  [unwired: 1 in, 6 out]
        n299 = call "首页显示设置.vi"() -> ()  [unwired: 12 in]
      }
      event "短信报警设置": Value Change {
        n300 = event-data() -> ()  [unwired: 1 in, 6 out]
        n301 = invoke class="VI" method="FP.Open"(reference=w428, "Activate"=TRUE ("激活？"), "State"=T14."Standard" ("状态")) -> ()  [unwired: 2 in, 5 out]
      }
      event "布尔": Mouse Down {
        n302 = event-data() -> ("CtlRef"=w430:refnum<vi>)  [unwired: 1 in, 6 out]
        n303 = property class="Bool (严格)"(reference=w430) -> ("Value"=w429:bool)  [unwired: 1 in, 2 out]
        n304 = case shown="假" w429 {
          tunnel: [w432 _] -> w431
          frame False {
            n305 = call "数字密码键盘.vi"() -> ("NewNumber"=w432:sgl)  [unwired: 1 in]
          }
          frame True {
          }
        }
        n306 = local write "输入密码"(w431) -> ()
      }
      event "微信关注设置": Value Change {
        n307 = event-data() -> ()  [unwired: 1 in, 6 out]
        n308 = global read "短信服务全局变量.vi" "站点"() -> (w433:string)
        n309 = call "创建参数二维码.vi"("站点"=w433) -> ()  [unwired: 11 in]
      }
    }
  }
  n310 = local write "开机启动"(w57) -> ()
  n311 = call <vilib>:"Close Config Data.vi"("error in (no error)"=w43, "refnum"=w40) -> ("error out"=w39:errorcluster)  [unwired: 8 in, 1 out]
  n312 = while {
    tunnel: w52 -> [w445]
    tunnel: w47 -> [_]
    tunnel: w39 -> [_]
    stop <- FALSE stop-if-true
    n313 = global read "副屏设置全局变量.vi" "启用副屏"() -> (w443:bool)
    n314 = global read "系统设置全局变量.vi" "时间阈值"() -> (w434:u16)
    n315 = global read "系统设置全局变量.vi" "流量阈值"() -> (w435:dbl)
    n316 = global read "系统设置全局变量.vi" "周期设置"() -> (w438:enum16{"自由设定", "国标协议", "流量设定"})
    n317 = global read "系统设置全局变量.vi" "运行间隔"() -> (w437:i16)
    n318 = global read "系统设置全局变量.vi" "运行模式"() -> (w436:enum16{"维护模式", "常规模式", "应急模式", "质控模式"})
    n319 = property class="VI"(reference=w445) -> (reference out=w442:refnum<vi>, "Exec.State"=w444:T7)  [unwired: 1 in, 1 out]
    n320 = Wait (ms)(milliseconds to wait=u32 1000 ("等待时间（毫秒）")) -> ()  [unwired: 1 out]
    n321 = global read "系统设置全局变量.vi" "自动运行启动参数"() -> (w446:T15)
    n322 = global read "系统设置全局变量.vi" "质控启动日期"() -> (w441:string)
    n323 = global read "系统设置全局变量.vi" "跨度核查时间"() -> (w439:u16)
    n324 = global read "系统设置全局变量.vi" "空白核查时间"() -> (w440:u16)
    n325 = global read "系统设置全局变量.vi" "24H周期设置"() -> (w447:bool[])
    n326 = case shown="\"Idle\"" w444 {
      tunnel: w443 -> [_ w450 w458]
      tunnel: w442 -> [_ w451 w459]
      frame "Bad", Default {
      }
      frame "Idle" {
        n327 = case shown="假" w450 {
          tunnel: w451 -> [_ w457]
          frame False {
          }
          frame True {
            n328 = invoke class="VI" method="Run VI"(reference=w457, "Wait until done"=FALSE ("结束前等待"), "Auto Dispose Ref"=FALSE ("自动销毁引用")) -> (reference out=w452:refnum<vi>)  [unwired: 2 in, 4 out]
            n329 = invoke class="VI" method="FP.Open"(reference=w452, "Activate"=TRUE ("激活？"), "State"=T14."Standard" ("状态")) -> ()  [unwired: 2 in, 5 out]
          }
        }
      }
      frame "Run top level" {
        n330 = case shown="假" w458 {
          tunnel: w459 -> [w460 _]
          frame False {
            n331 = invoke class="VI" method="Abort VI"(reference=w460) -> (reference out=w461:refnum<vi>)  [unwired: 2 in, 2 out]
            n332 = invoke class="VI" method="FP.Close"(reference=w461) -> ()  [unwired: 2 in, 3 out]
          }
          frame True {
          }
        }
      }
    }
    n333 = local write "时间阈值"(w434) -> ()
    n334 = local write "流量阈值"(w435) -> ()
    n335 = local write "周期设置"(w438) -> ()
    n336 = local write "运行间隔"(w437) -> ()
    n337 = local write "运行模式"(w436) -> ()
    n338 = local write "质控启动日期"(w441) -> ()
    n339 = local write "跨度核查时间"(w439) -> ()
    n340 = local write "空白核查时间"(w440) -> ()
    n341 = local write "24H周期设置"(w447) -> ()
    n342 = local write "自动运行启动参数"(w446) -> ()
  }
  n343 = call "Create balloon 队列.vi"() -> ("队列输出"=w1:refnum<queue>)  [unwired: 11 in]
  n344 = call <userlib>:"Initialize Balloon Engine.vi"("Balloon Direction"=enum16{"Top", "Bottom"}."Bottom" ("Balloon Position")) -> ("error out"=w3:errorcluster, "SmartBalloon Library.lvclass"=w6:refnum<class "SmartBalloon Library.lvclass">)  [unwired: 9 in]
  n345 = while {
    tunnel: w6 -> [w470]
    tunnel: [w469] -> w5
    tunnel: [w467] -> w4
    tunnel: w3 -> [w468]
    tunnel: w1 -> [w462]
    stop <- FALSE stop-if-true
    # "气球通知"
    n346 = Dequeue Element(queue=w462) -> (element=w463:cluster{"Title":string, "Body":string})  [unwired: 2 in, 3 out]
    n347 = flat-sequence {
      tunnel: w468 -> [w478]
      tunnel: [w477] -> w465
      tunnel: [w475] -> w464
      tunnel: w463 -> [w474]
      frame #0 {
        n348 = global read "短信服务全局变量.vi" "站点"() -> (w473:string)
        n349 = Unbundle By Name(w474) -> ("Title"=w472:string, "Body"=w471:string)
        n350 = call "消息推送.vi"("分析"=w471, "内容"=w472, "站点"=w473) -> ()  [unwired: 8 in, 1 out]
        n351 = call-poly <userlib>:"Initialize Balloon.vi"("Aesthetics"=T16 {"Colors"={"Font Color"=16777215, "Panel Color"=16749312}, "Display Time (ms)"=3000}, "error in (no error)"=w478, "Body"=w471, "Title"=w472) -> ("error out"=w475:errorcluster, "Balloon out"=w477:refnum<class "Text Balloon.lvclass">)  [unwired: 6 in]
      }
    }
    n352 = call <userlib>:"Add Balloon.vi"("error in (no error)"=w464, "Next Balloon"=w465, "SmartBalloon Engine Reference"=w470) -> ("error out"=w467:errorcluster, "SmartBalloon Engine Reference out"=w469:refnum<class "SmartBalloon Library.lvclass">)  [unwired: 7 in]
  }
  n353 = local write "updateconfiguration"(w8) -> ()
  n354 = global write "update全局.vi" "updateconfiguration"(w8) -> ()
  n355 = while {
    tunnel: [w479] -> _
    tunnel: w22 -> [_]
    stop <- FALSE stop-if-true
    n356 = event shown="[2] \"更新\": 值改变" {
      selector: _ -> [_ _ _]
      dyn-events: _ -> [_ _ _]
      timeout: 1000 -> [_ _ _]
      tunnel: [_ w490 _] -> w479
      event Timeout {
        n357 = event-data() -> ()  [unwired: 1 in, 3 out]
        n358 = local read "updateconfiguration"() -> (w482:T1)
        n359 = global write "update全局.vi" "updateconfiguration"(w482) -> ()
      }
      event "updateconfiguration": Value Change {
        n360 = event-data() -> ()  [unwired: 1 in, 6 out]
        n361 = Build Array("主机" ("section"), "用户" ("section"), "密码" ("key"), "远程路径" ("key"), "下载文件名" ("key"), "软件版本" ("key")) -> (w483:string[])
        n362 = call <vilib>:"Application Directory.vi"() -> ("Application Directory"=w493:path)
        n363 = Build Path(base path=w493, name or relative path="update\\data\\set.ini" ("名称或相对路径")) -> (appended path=w491:path)
        n364 = call "配置文件write.vi"("configuration file path"=w491, "键数组"=w483, "段"="应用程序交互" ("section")) -> ("error out"=w490:errorcluster)  [unwired: 8 in]
      }
      event "更新": Value Change {
        n365 = event-data() -> ()  [unwired: 1 in, 6 out]
        n366 = call "FTP自动升级更新main.vi"() -> ()  [unwired: 12 in]
      }
    }
  }
  n367 = call <userlib>:"Abort Balloon Engine.vi"("error in (no error)"=w4, "SmartBalloon Engine Reference"=w5) -> ("error out"=w2:errorcluster)  [unwired: 9 in]
  n368 = call <vilib>:"Simple Error Handler.vi"("error in (no error)"=w2) -> ()  [unwired: 4 in, 5 out]
